vi "Set up System Tray.vi"(5 "Icon Tip Strip Text":string, 7 "Image Path":path, 8 "error in":errorcluster, 11 "NotifyIcon in":refnum<class "NotifyIcon.lvclass">) -> (0 "error out":errorcluster, 3 "NotifyIcon out":refnum<class "NotifyIcon.lvclass">)   [LabVIEW 2014]
doc: "<B>Copyright</B>: (c) 2015 Ehsan Peymani. All rights reserved.\n\nThis subVI sets up the icon for system tray, make it invisible, and sets the tipstrip for tray icon."
uses:
  <userlib>/Notify Icon/Public/NotifyIcon.lvclass
  <userlib>/Notify Icon/Public/Tray Icon/Poly Set Methods VIs/Set Tray Icon (file).vi
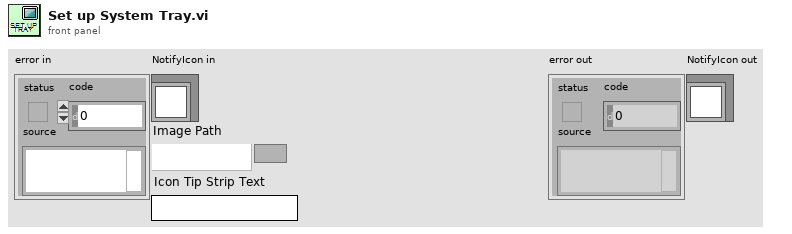
[diagram p1: front panel]
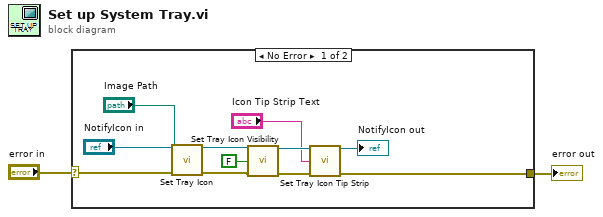
[diagram p0: block diagram]
diagram:
  n1 = case shown="No Error" "error in" {
    selector: "error in" -> [w8 w14]
    tunnel: [w7 w14] -> w1
    frame No Error {
      n2 = call-poly <userlib>:"Set Tray Icon.vi"("NotifyIcon in"="NotifyIcon in", "Image file"="Image Path", "error in (no error)"=w8) -> ("NotifyIcon out"=w13:refnum<class "NotifyIcon.lvclass">, "error out"=w12:errorcluster)  [unwired: 11 out]
      n3 = call <userlib>:"Set Tray Icon Visibility.vi"("NotifyIcon in"=w13, "Show Tray Icon"=FALSE, "error in (no error)"=w12) -> ("NotifyIcon out"=w10:refnum<class "NotifyIcon.lvclass">, "error out"=w9:errorcluster)  [unwired: 11 out]
      n4 = call <userlib>:"Set Tray Icon Tip Strip.vi"("NotifyIcon in"=w10, "Icon Tip Strip Text"="Icon Tip Strip Text", "error in (no error)"=w9) -> ("NotifyIcon out"=→"NotifyIcon out":refnum<class "NotifyIcon.lvclass">, "error out"=w7:errorcluster)  [unwired: 11 out]
    }
    frame Error {
    }
  }
  "error out" <- w1
